vi "0_WF_Anomaly_Detection(Dataset_Generation).vi"() -> ()   [LabVIEW 2020]
uses:
  Controls/Sampling_Info.ctl
  <vilib>/Utility/file.llb/Write Delimited Spreadsheet (DBL).vi
panel:
  in  "Dataset Folder Names":path[](array[path])=[path "Train", path "Test", path "Validation"]
  in  "# of Samples":i32[][](array[numeric])=[[10000, 0], [500, 500], [500, 500]]
  in  "Abnormal":string="Abnormal"
  in  "Normal":string="Normal"
  in  "General path":path=path "D:/working/Anomaly Detection"
  in  "Sampling Info":T1={"Fs"=10000.0, "#s"=2000.0}
  # "Overview: This VI generates synthetic Train, Test and Validation Datasets.\nThis project requires the last version of the DeepLTK toolkit\nToolkit:https://www.ngene.co/deep-learning-toolkit-for-labview \nInstructions:\n1. Specify the general path, where you want to generate the datasets.\n2. Specify the number of Normal and Abnormal samples in each dataset (Train, Validation and Test)\n3. Run the VI and observe generated dataset in your specified folder."
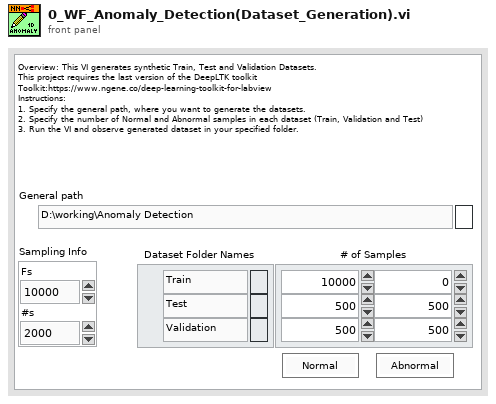
[diagram p1: front panel]
types:
  T1 = typedef "Sampling_Info.ctl" = cluster{"Fs":dbl, "#s":dbl}
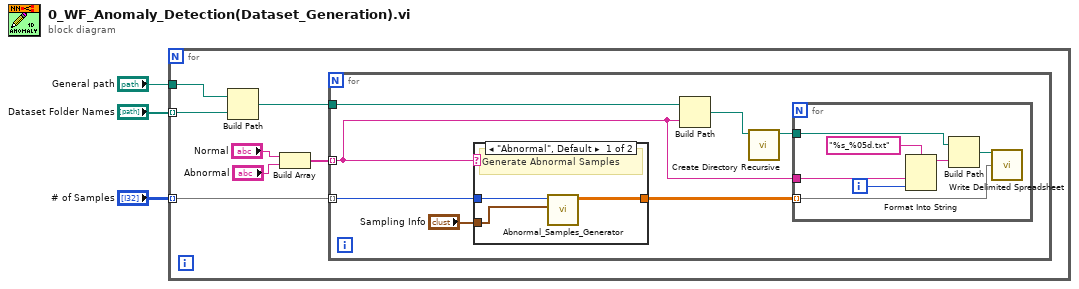
[diagram p0: block diagram]
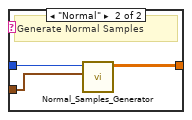
[diagram p2: hidden frame]
diagram:
  n1 = for {
    tunnel: "General path" -> [w10]
    tunnel: "Dataset Folder Names" -> [w9] mode=indexing
    tunnel: "# of Samples" -> [w4] mode=indexing
    n2 = Build Path(base path=w10, name or relative path=w9) -> (appended path=w6:path)
    n3 = Build Array("Normal", "Abnormal") -> (w5:string[])
    n4 = for {
      tunnel: w6 -> [w17]
      tunnel: w5 -> [w11] mode=indexing
      tunnel: w4 -> [w16] mode=indexing
      n5 = case shown="\"Abnormal\", Default" w11 {
        tunnel: w16 -> [w20 w23]
        tunnel: "Sampling Info" -> [w19 w22]
        tunnel: [w18 w21] -> w12
        frame "Abnormal", Default {
          # "Generate Abnormal Samples"
          n6 = call "Abnormal_Samples_Generator.vi"("Sampling Info"=w19, "Number of Abnormal Samples"=w20) -> ("Abnormal Samples"=w18:sgl[][])  [unwired: 9 in]
        }
        frame "Normal" {
          # "Generate Normal Samples"
          n7 = call "Normal_Samples_Generator.vi"("Sampling Info in"=w22, "Number of Normal Samples"=w23) -> ("data"=w21:sgl[][])  [unwired: 9 in]
        }
      }
      n8 = Build Path(base path=w17, name or relative path=w11) -> (appended path=w13:path)
      n9 = call <vilib>:"Create Directory Recursive.vi"("directory"=w13) -> ("directory copy"=w14:path)  [unwired: 4 in, 2 out]
      n10 = for {
        tunnel: w12 -> [w29] mode=indexing
        tunnel: w14 -> [w30]
        tunnel: w11 -> [w24]
        i -> [w25]
        n11 = Format Into String(format string="%s_%05d.txt", w24, w25) -> (resulting string=w26:string)  [unwired: 2 in, 1 out]
        n12 = Build Path(base path=w30, name or relative path=w26) -> (appended path=w28:path)
        n13 = call-poly <vilib>:"Write Delimited Spreadsheet.vi"("file path (dialog if empty)"=w28, "1D data"=w29) -> ()  [unwired: 12 in, 2 out]
      }
    }
  }
